vi "IO_FlagGB.vi"() -> ()   [LabVIEW 2019]
panel:
  in  "Life RecordQue":refnum<queue>
  out "exist":refnum<vi>
  in  "IO_Flag":T1[](array[typedef])
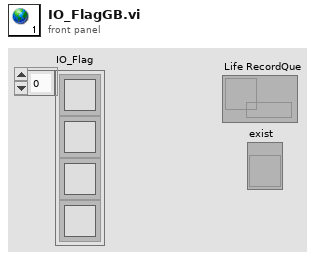
[diagram p1: front panel]
types:
  T1 = typedef "Semaphore RefNum" = refnum<k1>
diagram:
